vi "Auto_Routine_StraightThreePieceLeftNoteTRAJ.vi"(8 "error in (no error)":errorcluster) -> (0 "error out":errorcluster)   [LabVIEW 2023]
uses:
  Trajectory/TrajectoryGlobals.vi
  <vilib>/Rock Robotics/WPI/ThirdParty/JAS_Junk/TrajLib/Trajectory_Library.lvlib
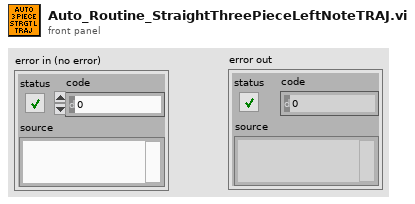
[diagram p1: front panel]
types:
  T1 = typedef "Trajectory_Library.lvlib/TRAJECTORY.ctl" = cluster{"TotalTImeSecs":dbl, "States":T2[]}
  T2 = typedef "Trajectory_Library.lvlib/TRAJ_STATE.ctl" = cluster{"TimeSeconds":dbl, "Velocity":dbl, "Acceleration":dbl, "POSE":T3, "Curvature":dbl}
  T3 = typedef "Trajectory_Library.lvlib/POSE2D.ctl" = cluster{"TRANSLATION":T4, "ROTATION":T5}
  T4 = typedef "Trajectory_Library.lvlib/TRANSLATION2D.ctl" = cluster{"X":dbl, "Y":dbl}
  T5 = typedef "Trajectory_Library.lvlib/ROTATION2D.ctl" = cluster{"VALUE":dbl, "COS":dbl, "SIN":dbl}
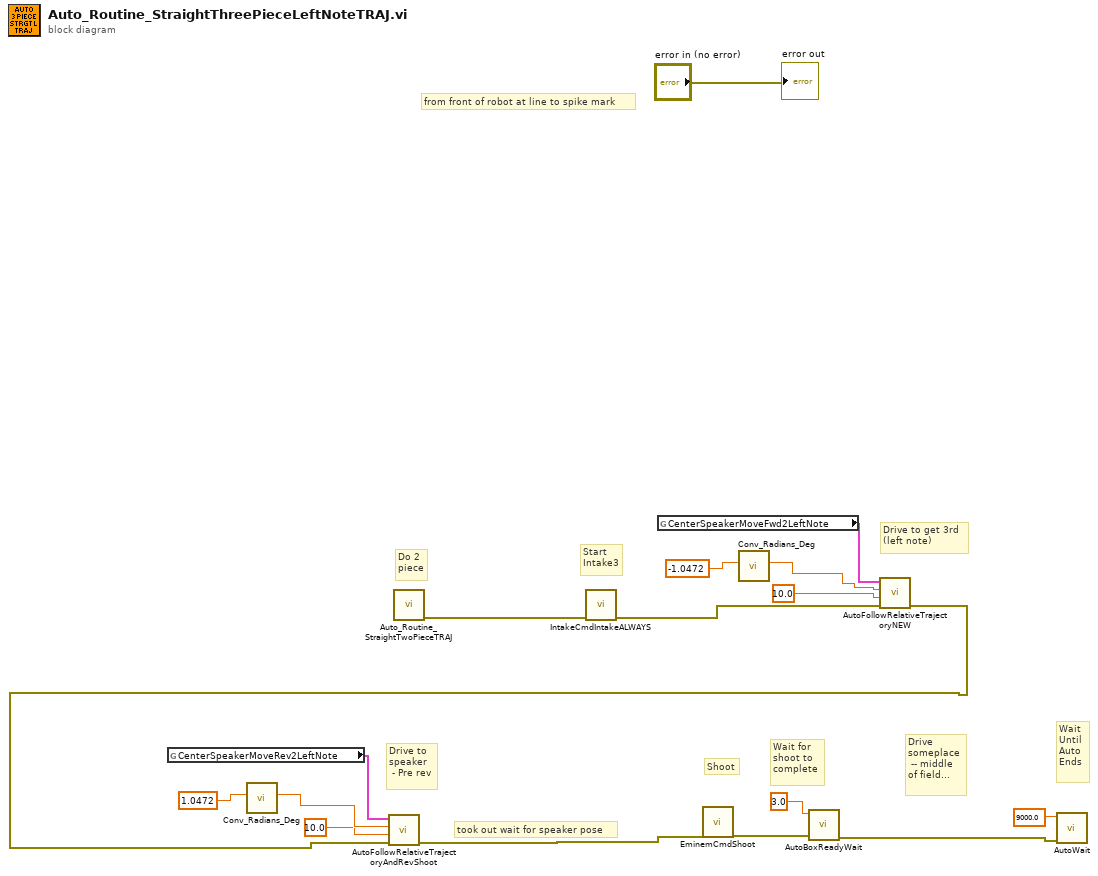
[diagram p0: block diagram]
diagram:
  # "Start\nIntake3"
  # "took out wait for speaker pose"
  # "Drive to get 3rd \n(left note)"
  # "Do 2 \npiece"
  # "Drive\nsomeplace\n -- middle\nof field..."
  # "Wait for\nshoot to\ncomplete"
  # "Shoot"
  # "Drive to\nspeaker\n - Pre rev"
  # "Wait\nUntil\nAuto \nEnds"
  # "from front of robot at line to spike mark"
  n1 = global read "TrajectoryGlobals.vi" "CenterSpeakerMoveRev2LeftNote"() -> (w10:T1)
  n2 = call <vilib>:"Conv_Radians_Deg.vi"("Radians"=1.0472) -> ("Degrees"=w8:dbl)  [unwired: 10 in]
  n3 = call "Auto_Routine_StraightTwoPieceTRAJ.vi"() -> ("error out"=w2:errorcluster)  [unwired: 11 in]
  n4 = call "IntakeCmdIntakeALWAYS.vi"("error in (no error)"=w2) -> ("error out"=w1:errorcluster)  [unwired: 10 in]
  n5 = global read "TrajectoryGlobals.vi" "CenterSpeakerMoveFwd2LeftNote"() -> (w15:T1)
  n6 = call <vilib>:"Conv_Radians_Deg.vi"("Radians"=-1.0472) -> ("Degrees"=w5:dbl)  [unwired: 10 in]
  n7 = call "AutoFollowRelativeTrajectoryNEW.vi"("error in (no error)"=w1, "TimeOut (s)"=10.0, "End Orientation"=w5, "Trajectory"=w15) -> ("error out"=w3:errorcluster)  [unwired: 7 in]
  n8 = call "AutoFollowRelativeTrajectoryAndRevShoot.vi"("error in (no error)"=w3, "TimeOut (s)"=10.0, "End Orientation"=w8, "Trajectory"=w10) -> ("error out"=w4:errorcluster)  [unwired: 7 in]
  n9 = call "EminemCmdShoot.vi"("error in (no error)"=w4) -> ("error out"=w12:errorcluster)  [unwired: 10 in]
  n10 = call "AutoBoxReadyWait.vi"("error in (no error)"=w12, "TimeOut (s)"=3.0) -> ("error out"=w11:errorcluster)  [unwired: 9 in]
  n11 = call "AutoWait.vi"("error in (no error)"=w11, "TimeOut (s)"=9000.0) -> ()  [unwired: 9 in, 1 out]
  "error out" <- "error in (no error)"
